vi "Analysis.vi"(8 "error in (no error)":errorcluster) -> (0 "error out":errorcluster)   [LabVIEW 2019]
uses:
  <vilib>/Utility/miscctls.llb/LVCursorListTypeDef.ctl
  <vilib>/Waveform/WDTOps.llb/WDT Get Waveform Subset DBL.vi
  <vilib>/measure/matone.llb/Extract Single Tone Information 1 Chan.vi
  <vilib>/measure/NI_MAPro.lvlib
panel:
  out "Acoustic Graph":T1(graph)
  in  "Mark Section Button":bool
  in  "Home Button":bool
  out "Selected File":path
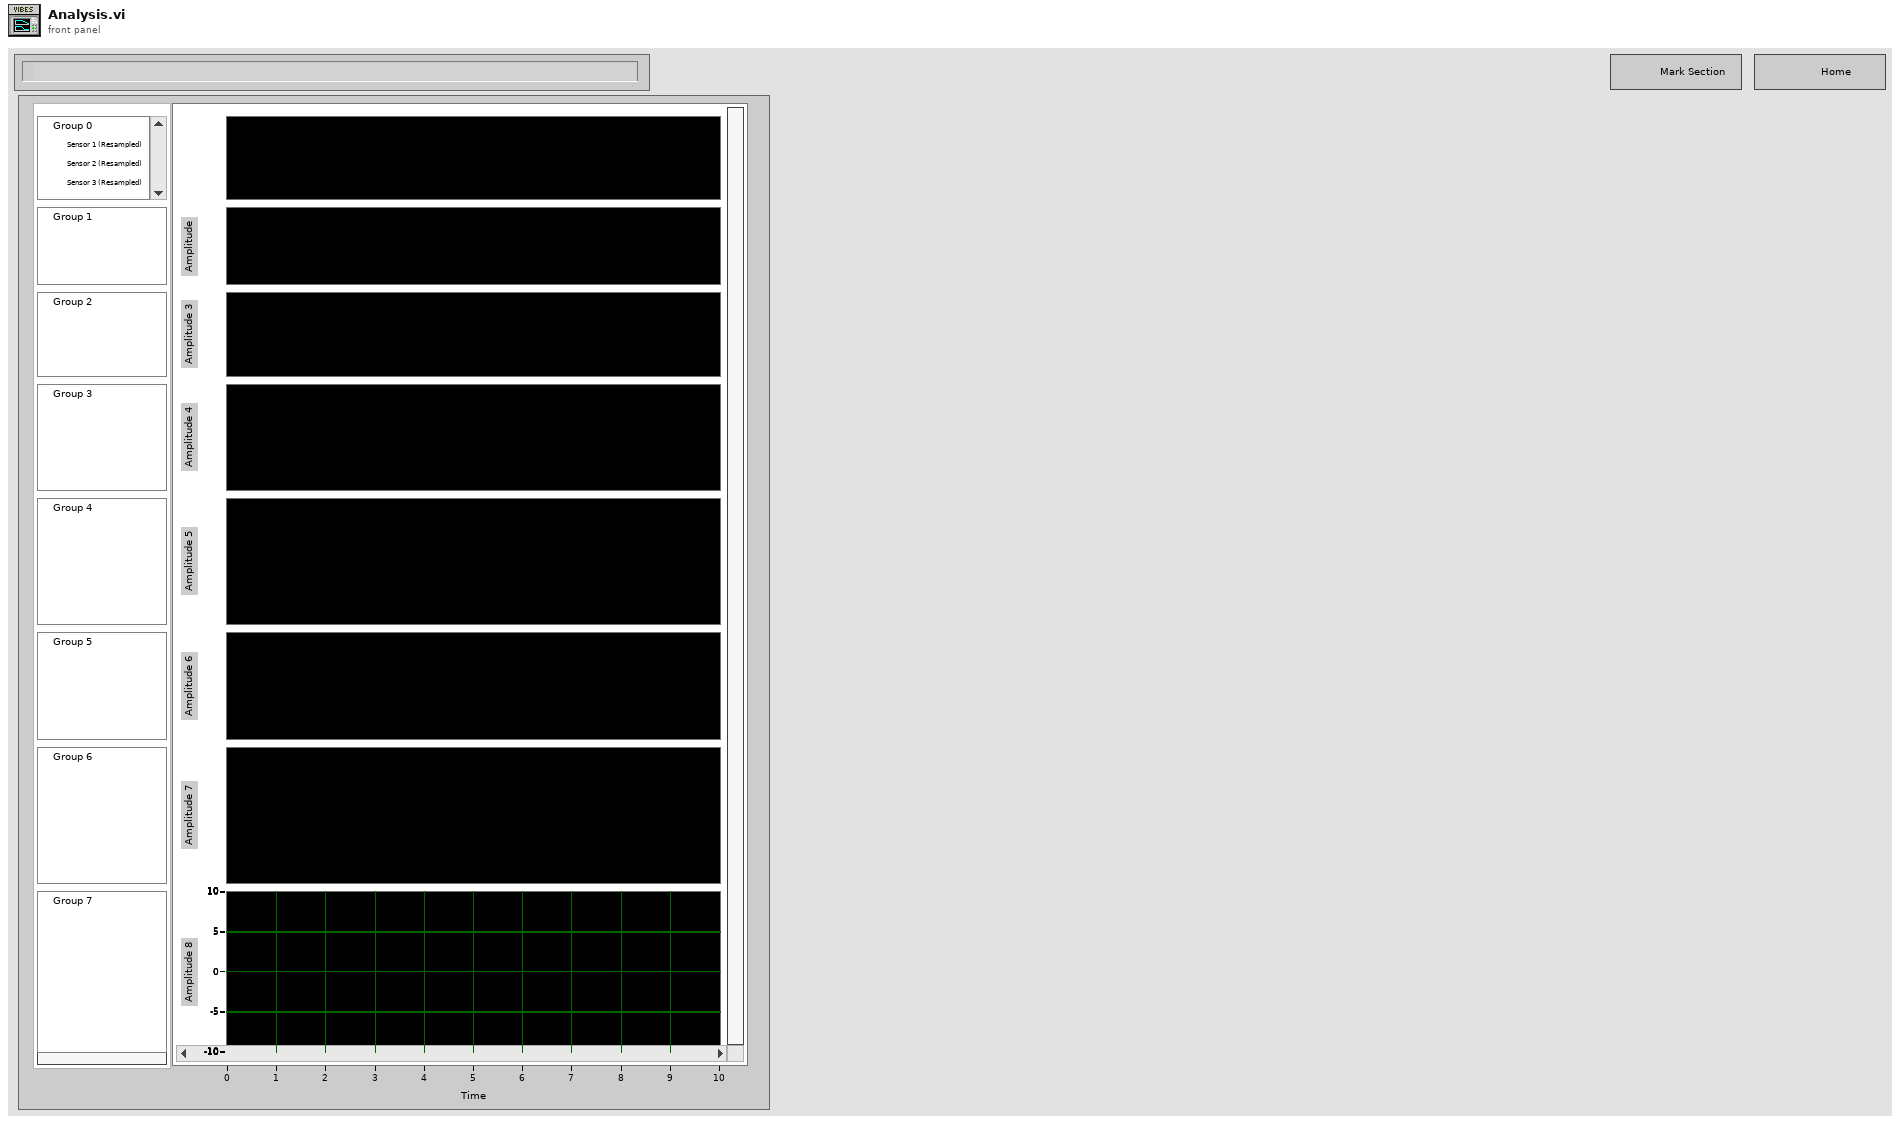
[diagram p1: front panel]
types:
  T1 = cluster{"Array of Waveform[0]":waveform(dbl), "Array of Waveform[1]":waveform(dbl), "Array of Waveform[2]":waveform(dbl), "Array of Waveform[3]":waveform(dbl), "Array of Waveform[4]":waveform(dbl), "Array of Waveform[5]":waveform(dbl), "Array of Waveform[6]":waveform(dbl), "Array of Waveform[7]":waveform(dbl), "Array of Waveform[8]":waveform(dbl)}
  T2 = typedef "LVCursorListTypeDef.ctl" = cluster{"Name":string, "Color":u32, "Style":u8, "Point Style":u8, "Name Visible":bool, "Allow Drag":bool, "Cursor Mode":u32, "Plot":i32, "Index":i32, "Position":cluster{"X":dbl, "Y":dbl}, "X Scale":u32, "Y Scale":u32, "Watch Plots":i32[], "Watch All Plots":bool, "Plot Area":i32, "Label Offset":cluster{"X":dbl, "Y":dbl}}[]
  T3 = enum16{"open", "replace", "create", "open or create", "replace or create", "replace or create with confirmation"}
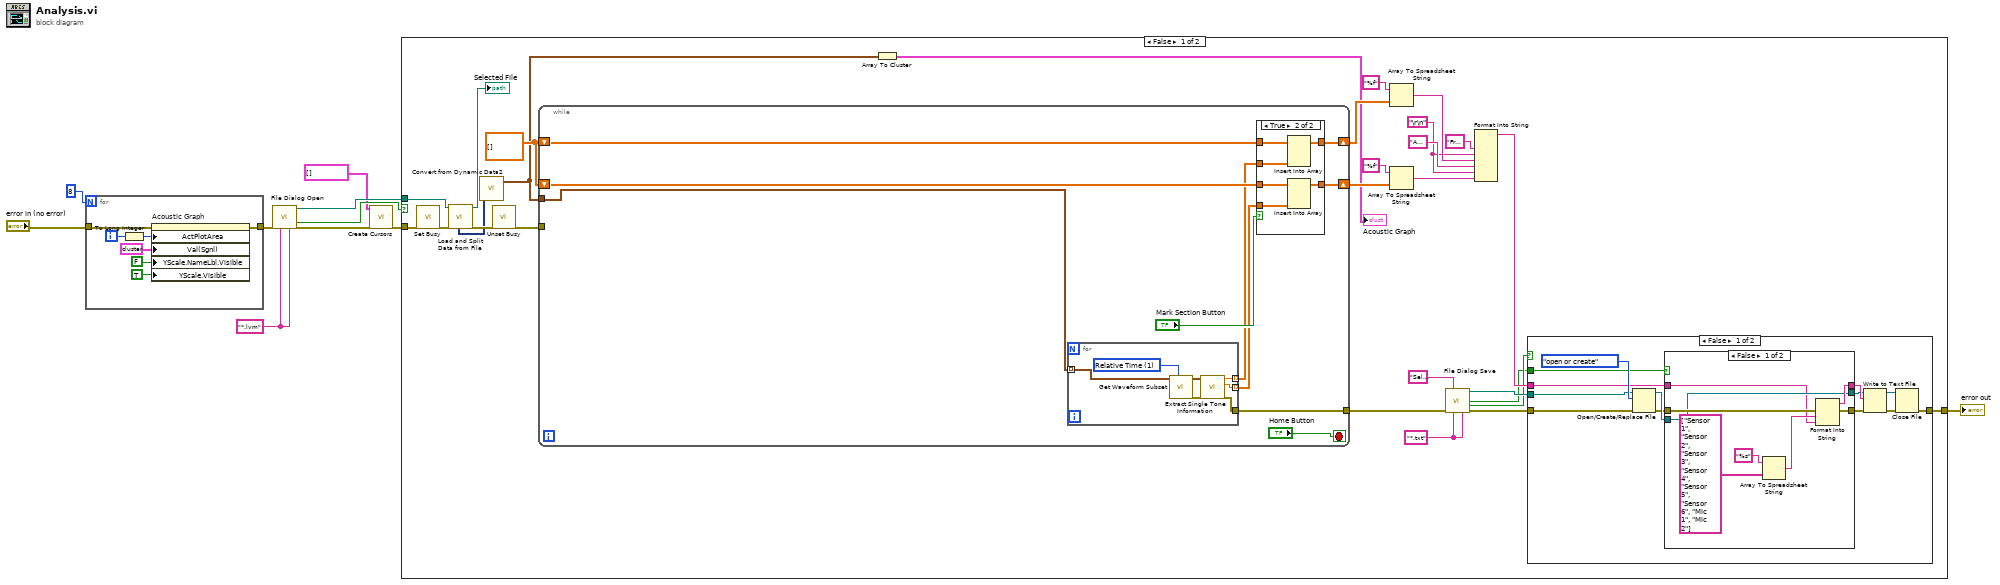
[diagram p0: block diagram]
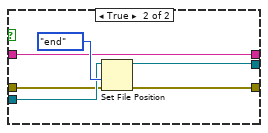
[diagram p2: hidden frame]
diagram:
  w8 = "*.lvm" ("pattern label")
  n1 = for {
    N: 8 -> [_]
    tunnel: "error in (no error)" -> [w16]
    tunnel: [w15] -> w1
    i -> [w14]
    n2 = To Long Integer(number=w14) -> (32bit integer=w13:i32)
    n3 = property on="Acoustic Graph" class="MixedGraph (strict)"(error in=w16, "ActPlotArea"=w13, "Val(Sgnl)"=T1 {"Array of Waveform[0]"={"t0"=timestamp(0 s since 1904-01-01), "dt"=1.0, "Y"=[]}, "Array of Waveform[1]"={"t0"=timestamp(0 s since 1904-01-01), "dt"=1.0, "Y"=[]}, "Array of Waveform[2]"={"t0"=timestamp(0 s since 1904-01-01), "dt"=1.0, "Y"=[]}, "Array of Waveform[3]"={"t0"=timestamp(0 s since 1904-01-01), "dt"=1.0, "Y"=[]}, "Array of Waveform[4]"={"t0"=timestamp(0 s since 1904-01-01), "dt"=1.0, "Y"=[]}, "Array of Waveform[5]"={"t0"=timestamp(0 s since 1904-01-01), "dt"=1.0, "Y"=[]}, "Array of Waveform[6]"={"t0"=timestamp(0 s since 1904-01-01), "dt"=1.0, "Y"=[]}, "Array of Waveform[7]"={"t0"=timestamp(0 s since 1904-01-01), "dt"=1.0, "Y"=[]}, "Array of Waveform[8]"={"t0"=timestamp(0 s since 1904-01-01), "dt"=1.0, "Y"=[]}} ("Value (Signaling)"), "YScale.NameLbl.Visible"=FALSE ("Y Scale.Visible"), "YScale.Visible"=TRUE ("Y Scale.Visible")) -> (error out=w15:errorcluster)  [unwired: 1 in, 1 out]
  }
  n4 = call "File Dialog Open"("error in"=w1, "pattern (all files)"=w8, "pattern label"=w8) -> ("selected path"=w9:path, "cancelled"=w10:bool, "error out"=w6:errorcluster)  [unwired: 9 in, 1 out]
  n5 = call "Create Cursors.vi"("Error In"=w6, "Cursor List"=T2 []) -> ("Error Out"=w2:errorcluster)  [unwired: 8 in, 1 out]
  n6 = case shown="False" w10 {
    tunnel: w2 -> [w43 w99]
    tunnel: w9 -> [w44 _]
    tunnel: [w35 w99] -> w5
    frame False {
      w22 = "*.txt" ("pattern label")
      w24 = "\r\n"
      w40 = dbl[][] [] ("Amplitudes")
      n7 = call <vilib>:"Set Busy.vi"("error in (no error)"=w43) -> ("error out"=w42:errorcluster)  [unwired: 9 in, 1 out]
      n8 = call "Load and Split Data from File.vi"("Filename"=w44, "Error In"=w42) -> ("All"=w20:dynamicdata, "Filename Out"=→"Selected File":path, "Error Out"=w39:errorcluster)  [unwired: 7 in, 8 out]
      n9 = call "Convert from Dynamic Data2"("Dynamic Data Type"=w20) -> ("Array of Waveform"=w19:waveform(dbl)[])  [unwired: 3 in]
      n10 = call <vilib>:"Unset Busy.vi"("error in (no error)"=w39) -> ("error out"=w41:errorcluster)  [unwired: 10 in]
      n11 = while {
        tunnel: w41 -> [_]
        tunnel: w19 -> [w82]
        shift-right: [w76] -> w34
        shift-left: w40 -> [w80]
        shift-right: [w75] -> w31
        shift-left: w40 -> [w79]
        tunnel: [w74] -> w38
        stop <- "Home Button" stop-if-true
        n12 = for {
          tunnel: w82 -> [w98] mode=indexing
          tunnel: [w96] -> w78 mode=indexing
          tunnel: [w95] -> w77 mode=indexing
          tunnel: [w92] -> w74
          w94 = u16 1 items=["Samples", "Relative Time"] ("start/duration format")
          n13 = call-poly <vilib>:"Get Waveform Subset.vi"("start/duration format"=w94, "waveform in"=w98) -> ("error out"=w93:errorcluster, "waveform out"=w97:waveform(dbl))  [unwired: 4 in, 2 out]
          n14 = call-poly <vilib>:"Extract Single Tone Information.vi"("error in (no error)"=w93, "time signal in"=w97) -> ("error out"=w92:errorcluster, "detected amplitude"=w95:dbl, "detected frequency"=w96:dbl)  [unwired: 4 in, 3 out]
        }
        n15 = case shown="True" "Mark Section Button" {
          tunnel: w80 -> [w85 w91]
          tunnel: w79 -> [w84 w90]
          tunnel: w78 -> [_ w89]
          tunnel: w77 -> [_ w88]
          tunnel: [w85 w87] -> w76
          tunnel: [w84 w86] -> w75
          frame False {
          }
          frame True {
            n16 = Insert Into Array(array=w91, new element=w89) -> (w87:dbl[][])  [unwired: 2 in]
            n17 = Insert Into Array(array=w90, new element=w88) -> (w86:dbl[][])  [unwired: 2 in]
          }
        }
      }
      n18 = Array To Cluster(array=w19) -> (cluster=→"Acoustic Graph":T1)
      n19 = Array To Spreadsheet String(array=w34, 3:"%f" ("format string")) -> (spreadsheet string=w26:string)  [unwired: 1 in]
      n20 = Array To Spreadsheet String(array=w31, 3:"%f" ("format string")) -> (spreadsheet string=w23:string)  [unwired: 1 in]
      n21 = call "File Dialog Save"("prompt"="Select a Save Location", "error in"=w38, "pattern (all files)"=w22, "pattern label"=w22) -> ("selected path"=w36:path, "exists"=w28:bool, "cancelled"=w29:bool, "error out"=w37:errorcluster)  [unwired: 8 in]
      n22 = Format Into String("Frequency Values" ("initial string"), w24, w26, "Amplitude Values", w24, w23) -> (resulting string=w30:string)  [unwired: 3 in, 1 out]
      n23 = case shown="False" w29 {
        tunnel: w37 -> [w58 w73]
        tunnel: w36 -> [w56 _]
        tunnel: [w53 w73] -> w35
        tunnel: w30 -> [w48 _]
        tunnel: w28 -> [w50 _]
        frame False {
          n24 = Open/Create/Replace File(file path (use dialog)=w56, error in=w58, operation (0:open)=T3."open or create") -> (refnum out=w52:refnum<file>, error out=w51:errorcluster)  [unwired: 3 in, 1 out]
          n25 = case shown="False" w50 {
            tunnel: w52 -> [w60 w71]
            tunnel: w51 -> [w66 w70]
            tunnel: [w65 w69] -> w49
            tunnel: w48 -> [w59 w68]
            tunnel: [w61 w68] -> w47
            tunnel: [w60 w67] -> w46
            frame False {
              n26 = Array To Spreadsheet String(array=string[] ["Sensor 1", "Sensor 2", "Sensor 3", "Sensor 4", "Sensor 5", "Sensor 6", "Mic 1", "Mic 2"], 3:"%s" ("format string")) -> (spreadsheet string=w62:string)  [unwired: 1 in]
              n27 = Format Into String(error in=w66, w62, w59) -> (resulting string=w61:string, error out=w65:errorcluster)  [unwired: 2 in]
            }
            frame True {
              n28 = Set File Position(refnum=w71, from (0:start)=enum16{"start", "end", "current"}."end", error in=w70) -> (refnum out=w67:refnum<file>, error out=w69:errorcluster)  [unwired: 1 in]
            }
          }
          n29 = Write to Text File(file (use dialog)=w46, text=w47, error in=w49) -> (refnum out=w54:refnum<file>, error out=w55:errorcluster)  [unwired: 1 in, 1 out]
          n30 = Close File(refnum=w54, error in=w55) -> (error out=w53:errorcluster)  [unwired: 1 out]
        }
        frame True {
        }
      }
    }
    frame True {
    }
  }
  "error out" <- w5
